vi "GPS Plot Obstacles from SICK.vi"(4 "Current GPS Coordinates":cluster{"Longitude":dbl, "Latitude":dbl}, 5 "SICK Array":i32[](array[numeric])) -> (1 "Array of Obstacle GPS":cluster{"Longitude":dbl, "Latitude":dbl}[](array[cluster]))   [LabVIEW 2009]
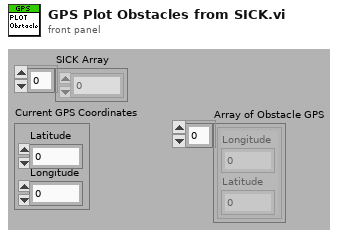
[diagram p1: front panel]
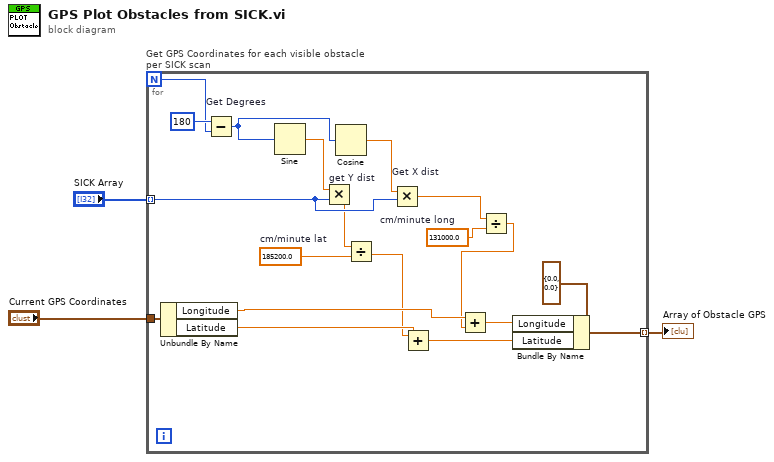
[diagram p0: block diagram]
diagram:
  n1 = for "Get GPS Coordinates for each visible obstacle per SICK scan" {
    N -> [w21]
    tunnel: "SICK Array" -> [w17] mode=indexing
    tunnel: "Current GPS Coordinates" -> [w16]
    tunnel: [w10] -> w1 mode=indexing
    w6 = 131000.0  # cm/minute long
    w9 = 185200.0  # cm/minute lat
    n2 = Unbundle By Name(w16) -> ("Longitude"=w14:dbl, "Latitude"=w15:dbl)
    n3 = Subtract "Get Degrees"(x=180, y=w21) -> (x-y=w20:i32)
    n4 = Sine(x=w20) -> (sin(x)=w19:dbl)
    n5 = Multiply "get Y dist"(x=w19, y=w17) -> (x*y=w8:dbl)
    n6 = Cosine(x=w20) -> (cos(x)=w18:dbl)
    n7 = Divide(x=w8, y=w9) -> (x/y=w7:dbl)
    n8 = Multiply "Get X dist"(x=w18, y=w17) -> (x*y=w5:dbl)
    n9 = Add(x=w7, y=w15) -> (x+y=w13:dbl)
    n10 = Divide(x=w5, y=w6) -> (x/y=w4:dbl)
    n11 = Add(x=w14, y=w4) -> (x+y=w12:dbl)
    n12 = Bundle By Name(cluster=cluster{"Longitude":dbl, "Latitude":dbl} {"Longitude"=0.0, "Latitude"=0.0} ("Current GPS Coordinates 2"), "Longitude"=w12, "Latitude"=w13) -> (w10:cluster{"Longitude":dbl, "Latitude":dbl})
  }
  "Array of Obstacle GPS" <- w1
